vi "Close.vi"(8 "error in":errorcluster, 11 "Yokogawa in":refnum<class "Yokogawa.lvclass">) -> (0 "error out":errorcluster, 3 "Yokogawa out":refnum<class "Yokogawa.lvclass">)   [LabVIEW 2015, in "Yokogawa.lvclass"]
uses:
  Yokogawa.lvclass
  Parent/Power Meter.lvclass/Power Meter.ctl
  Parent/Read Address.vi
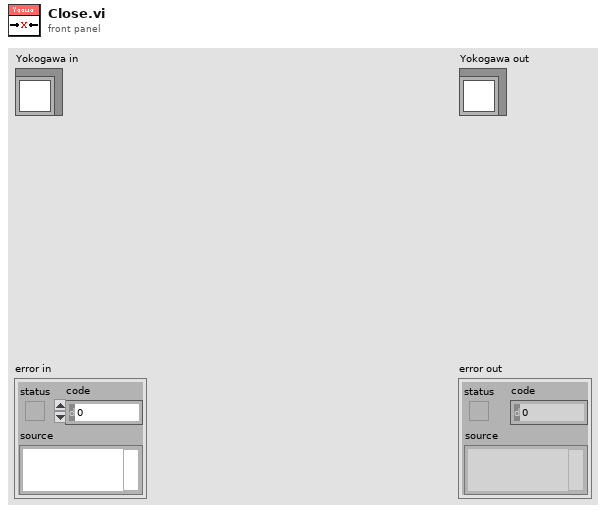
[diagram p1: front panel]
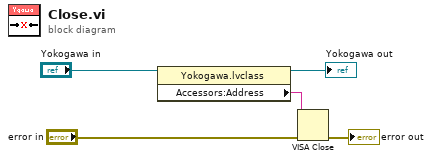
[diagram p0: block diagram]
diagram:
  n1 = property class="Yokogawa.lvclass"(reference="Yokogawa in") -> (reference out=→"Yokogawa out":refnum<class "Yokogawa.lvclass">, "Accessors:Address"=w4:string)  [unwired: 1 in, 1 out]
  n2 = VISA Close(VISA resource name=w4, error in (no error)="error in") -> (error out=→"error out":errorcluster)
